vi "helper-serial-log-to-string.vi"(10 "filter":T1={"Status"=0, "Date"="", "Caller"="", "Type"="", "IOname"="", "Calib"="", "Uncalib"="", "Vsdt"="Uncalib", "StatusMsg"=""}, 11 "input cluster":T2 {"IOnode"."calibration"."Y" format="%#.3f"; "IOnode"."calibration"."X" format="%#.3f"; "IOnode"."ADDR" format="%04d"}) -> (1 "output cluster":cluster{"Status":bool}, 2 "Snapshot":T1={"Status"=0, "Date"="", "Caller"="", "Type"="", "IOname"="", "Calib"="", "Uncalib"="", "Vsdt"="Uncalib", "StatusMsg"=""}, 3 "String":string)   [LabVIEW 2024]
uses:
  controls/cluster-com-log.ctl
  controls/IONode.ctl
  controls/type.address.ctl
  controls/enum.io.type.ctl
  controls/enum.io.mode.ctl
  controls/typeXyPoint.ctl
  controls/eng-serial-log.ctl
  <vilib>/Utility/error.llb/Trim Whitespace One-Sided.vi
panel:
  out "result":bool
  out "Name Found":bool
  out "Type Found":bool
  out "Caller Found":bool
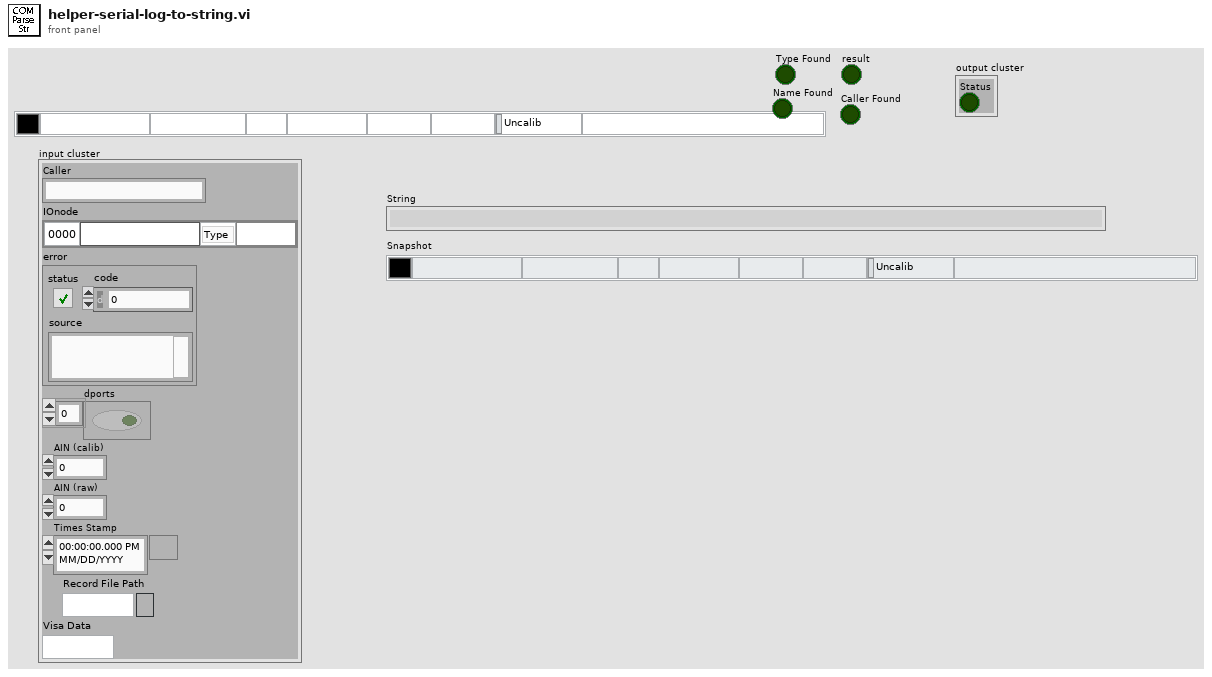
[diagram p1: front panel]
types:
  T1 = typedef "eng-serial-log.ctl" = cluster{"Status":u32, "Date":string, "Caller":string, "Type":string, "IOname":string, "Calib":string, "Uncalib":string, "Vsdt":string, "StatusMsg":string}
  T2 = typedef "cluster-com-log.ctl" = cluster{"Caller":string, "IOnode":T3, "error":errorcluster, "dports":bool[], "AIN (calib)":dbl, "AIN (raw)":u16, "Times Stamp":timestamp, "Record File Path":path, "Visa Data":string}
  T3 = typedef "IONode.ctl" = cluster{"ADDR":T4, "Label":string, "Type":T5, "Mode":T6, "Value":string, "Tags":string, "calibration":T7[]}
  T4 = typedef "type.address.ctl" = u16
  T5 = typedef "enum.io.type.ctl" = enum16{"Type", "DI", "DO", "AI", "AO", "VL", "BUF"}
  T6 = typedef "enum.io.mode.ctl" = enum16{"Mode", "RIO", "SIM"}
  T7 = typedef "typeXyPoint.ctl" = cluster{"X":dbl, "Y":dbl}
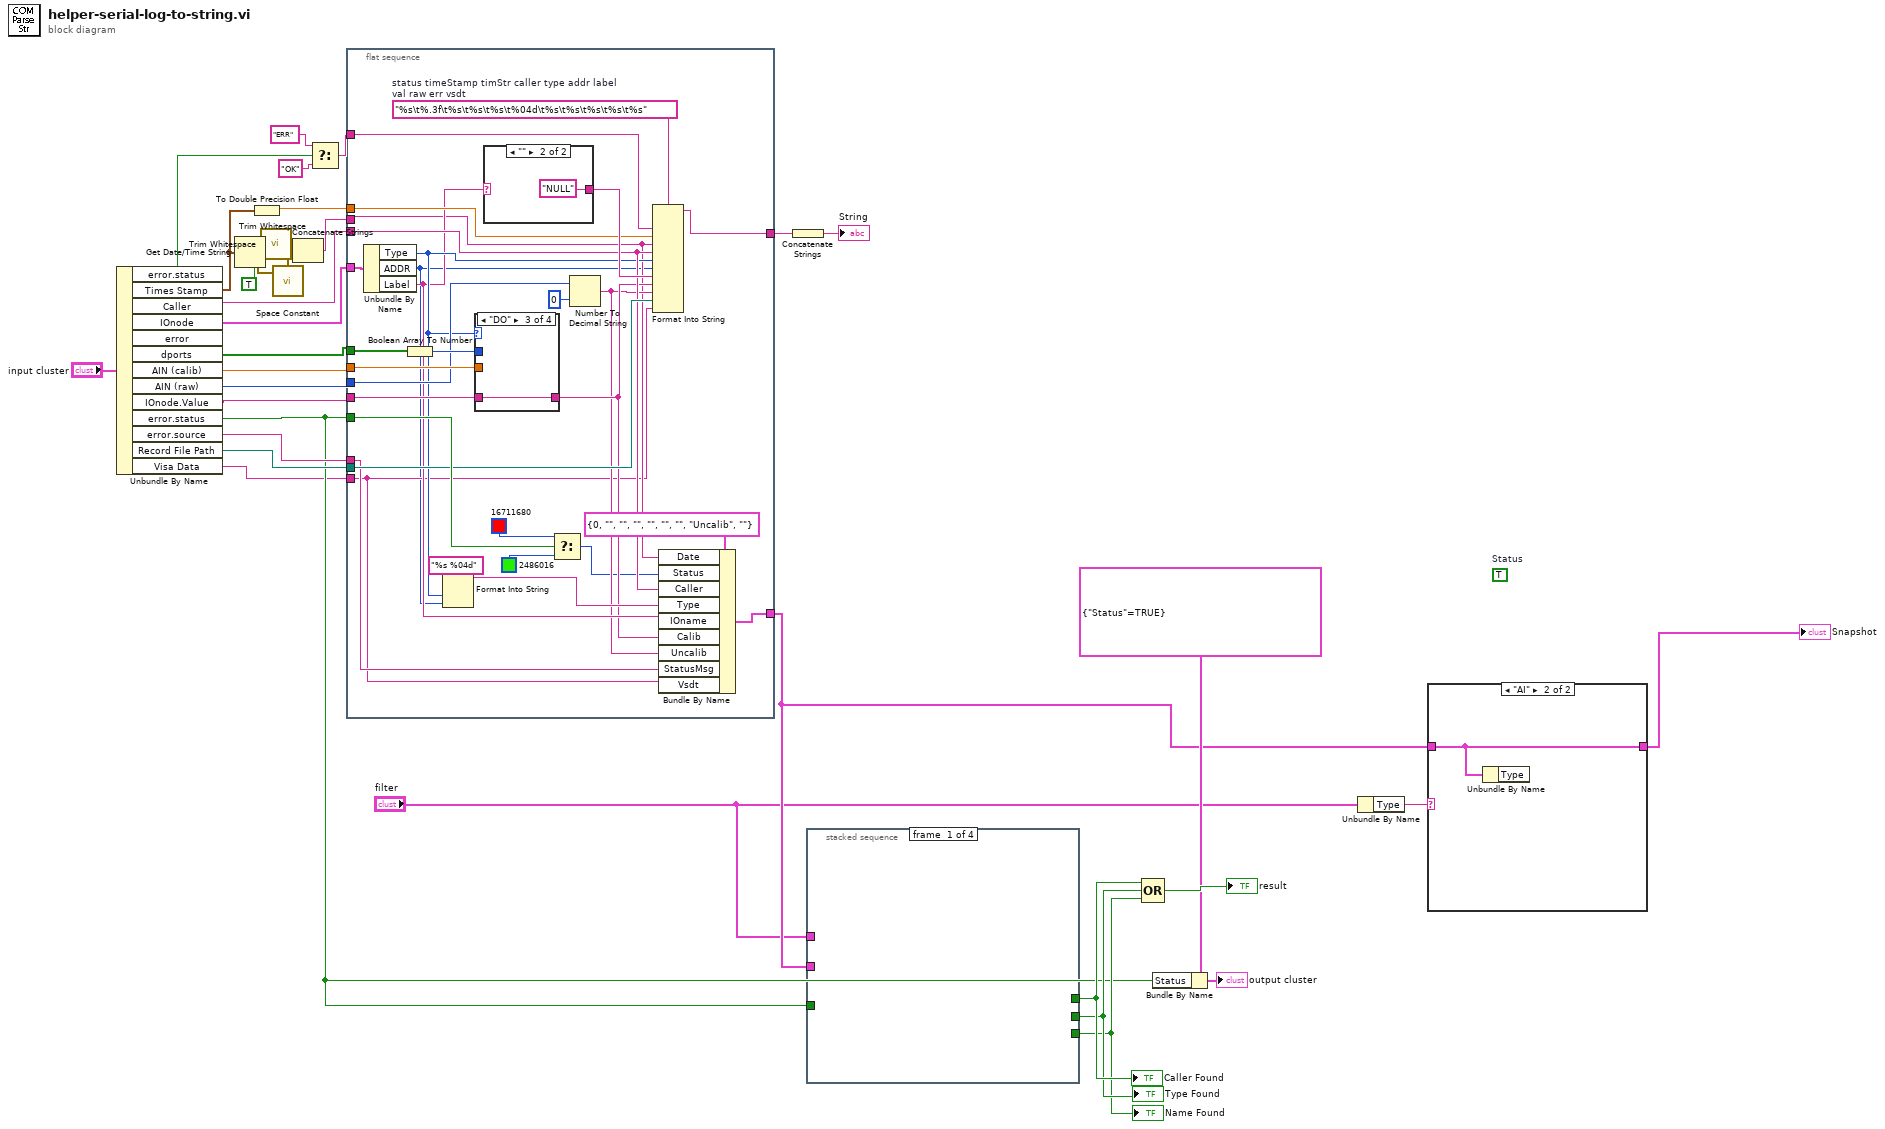
[diagram p0: block diagram]
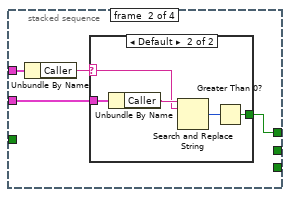
[diagram p3: hidden frame]
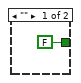
[diagram p4: hidden frame]
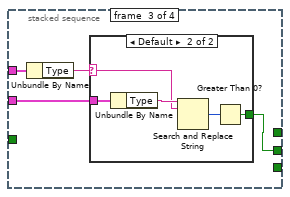
[diagram p5: hidden frame]
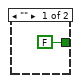
[diagram p6: hidden frame]
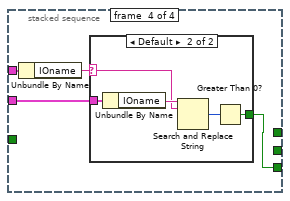
[diagram p7: hidden frame]
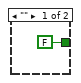
[diagram p8: hidden frame]
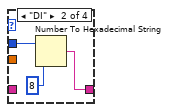
[diagram p11: hidden frame]
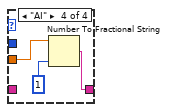
[diagram p12: hidden frame]
diagram:
  (unwired) TRUE  # Status
  n1 = Unbundle By Name("input cluster") -> ("error.status"=w17:bool, "Times Stamp"=w26:timestamp, "Caller"=w31:string, "IOnode"=w32:T3, "dports"=w35:bool[], "AIN (calib)"=w34:dbl, "AIN (raw)"=w33:u16, "IOnode.Value"=w36:string, "error.status"=w8:bool, "error.source"=w27:string, "Record File Path"=w19:path, "Visa Data"=w5:string)  [unwired: 1 out]
  n2 = Get Date/Time String(seconds (now)=w26, want seconds? (F)=TRUE) -> (date string=w24:string, time string=w23:string)  [unwired: 1 in]
  n3 = To Double Precision Float(number=w26) -> (double precision float=w20:dbl)
  n4 = call <vilib>:"Trim Whitespace.vi"("string"=w23) -> ("trimmed string"=w6:string)  [unwired: 1 in]
  n5 = call <vilib>:"Trim Whitespace.vi"("string"=w24) -> ("trimmed string"=w7:string)  [unwired: 1 in]
  n6 = call <vilib>:"Space Constant.vi"() -> ("String"=w22:string)
  n7 = Concatenate Strings(w7, w22, w6) -> (w21:string)
  n8 = Select(t="ERR" ("f"), s=w17, f="OK") -> (s? t:f=w15:string)
  n9 = flat-sequence {
    tunnel: w31 -> [w50]
    tunnel: w32 -> [w66]
    tunnel: [w65] -> w29
    tunnel: w35 -> [w63]
    tunnel: w34 -> [w61]
    tunnel: w8 -> [w60]
    tunnel: w36 -> [w58]
    tunnel: w33 -> [w57]
    tunnel: w27 -> [w43]
    tunnel: w21 -> [w44]
    tunnel: w20 -> [w55]
    tunnel: w19 -> [w54]
    tunnel: w15 -> [w53]
    tunnel: [w51] -> w4
    tunnel: w5 -> [w39]
    frame #0 {
      w64 = "%s\t%.3f\t%s\t%s\t%s\t%04d\t%s\t%s\t%s\t%s\t%s"  # status timeStamp timStr caller type addr label val raw err vsdt
      n10 = Unbundle By Name(w66) -> ("Type"=w49:T5, "ADDR"=w37:T4, "Label"=w47:string)
      n11 = Boolean Array To Number(Boolean array=w63) -> (number=w62:u32)
      n12 = Format Into String(format string="%s %04d", w49, w37) -> (resulting string=w48:string)  [unwired: 2 in, 1 out]
      n13 = case shown="\"DO\"" w49 {
        tunnel: [_ w70 w72 w74] -> w46
        tunnel: w62 -> [_ w71 _ _]
        tunnel: w61 -> [_ _ _ w75]
        tunnel: w58 -> [_ _ w72 _]
        frame Default {
        }
        frame "DI" {
          n14 = Number To Hexadecimal String(1:i16 8 ("width (-)"), 2:w71) -> (0:w70:string)
        }
        frame "DO" {
        }
        frame "AI" {
          n15 = Number To Fractional String(number=w75, precision (6)=i16 1) -> (F-format string=w74:string)  [unwired: 2 in]
        }
      }
      n16 = case shown="\"\"" w47 {
        selector: w47 -> [w67 _]
        tunnel: [w67 "NULL"] -> w59
        frame Default {
        }
        frame "" {
        }
      }
      n17 = Select(t=u32 16711680 ("Status"), s=w60, f=u32 2486016 ("Status")) -> (s? t:f=w42:u32)
      n18 = Number To Decimal String(number=w57, width (-)=i16 0) -> (decimal integer string=w45:string)
      n19 = Format Into String(format string=w64, w53, w55, w44, w50, w49, w37, w59, w46, w45, w54, w39) -> (resulting string=w65:string)  [unwired: 2 in, 1 out]
      n20 = Bundle By Name(cluster=T1 {"Status"=0, "Date"="", "Caller"="", "Type"="", "IOname"="", "Calib"="", "Uncalib"="", "Vsdt"="Uncalib", "StatusMsg"=""}, "Date"=w44, "Status"=w42, "Caller"=w50, "Type"=w48, "IOname"=w47, "Calib"=w46, "Uncalib"=w45, "StatusMsg"=w43, "Vsdt"=w39) -> (w51:T1)
    }
  }
  n21 = Concatenate Strings(w29) -> (→"String":string)
  n22 = stacked-sequence {
    tunnel: "filter" -> [_ w79 w89 w99]
    tunnel: w4 -> [_ w78 w88 w98]
    tunnel: [_ w76 _ _] -> w14
    tunnel: [_ _ w86 _] -> w13
    tunnel: [_ _ _ w96] -> w12
    tunnel: w8 -> [_ _ _ _]
    frame #0 {
    }
    frame #1 {
      n23 = Unbundle By Name(w79) -> ("Caller"=w77:string)
      n24 = case shown="Default" w77 {
        selector: w77 -> [_ w81]
        tunnel: w78 -> [_ w85]
        tunnel: [FALSE w82] -> w76
        frame "" {
        }
        frame Default {
          n25 = Unbundle By Name(w85) -> ("Caller"=w84:string)
          n26 = Search and Replace String(input string=w84, search string=w81) -> (number of replacements=w83:i32)  [unwired: 6 in, 3 out]
          n27 = Greater Than 0?(x=w83) -> (x > 0?=w82:bool)
        }
      }
    }
    frame #2 {
      n28 = Unbundle By Name(w89) -> ("Type"=w87:string)
      n29 = case shown="Default" w87 {
        selector: w87 -> [_ w91]
        tunnel: w88 -> [_ w95]
        tunnel: [FALSE w92] -> w86
        frame "" {
        }
        frame Default {
          n30 = Unbundle By Name(w95) -> ("Type"=w94:string)
          n31 = Search and Replace String(input string=w94, search string=w91) -> (number of replacements=w93:i32)  [unwired: 6 in, 3 out]
          n32 = Greater Than 0?(x=w93) -> (x > 0?=w92:bool)
        }
      }
    }
    frame #3 {
      n33 = Unbundle By Name(w99) -> ("IOname"=w97:string)
      n34 = case shown="Default" w97 {
        selector: w97 -> [_ w101]
        tunnel: w98 -> [_ w105]
        tunnel: [FALSE w102] -> w96
        frame "" {
        }
        frame Default {
          n35 = Unbundle By Name(w105) -> ("IOname"=w104:string)
          n36 = Search and Replace String(input string=w104, search string=w101) -> (number of replacements=w103:i32)  [unwired: 6 in, 3 out]
          n37 = Greater Than 0?(x=w103) -> (x > 0?=w102:bool)
        }
      }
    }
  }
  "Caller Found" <- w14
  "Type Found" <- w13
  "Name Found" <- w12
  n38 = Compound Arithmetic op=OR(w14, w13, w12) -> (→"result":bool)
  n39 = Bundle By Name(cluster=cluster{"Status":bool} {"Status"=TRUE}, "Status"=w8) -> (→"output cluster":cluster{"Status":bool})
  n40 = Unbundle By Name("filter") -> ("Type"=w1:string)
  n41 = case shown="\"AI\"" w1 {
    tunnel: w4 -> [w106 w107]
    tunnel: [w106 w107] -> w3
    frame "", Default {
    }
    frame "AI" {
      n42 = Unbundle By Name(w107) -> ()  [unwired: 1 out]
    }
  }
  "Snapshot" <- w3
